vi "Validate Meas Name in Library.vi"(0 "Path":path, 5 "library name":string, 11 "error in (no error)":errorcluster) -> (4 "found":bool, 15 "error out":errorcluster)   [LabVIEW 2021, in "Migrator.lvlib"]
uses:
  Migrator.lvlib
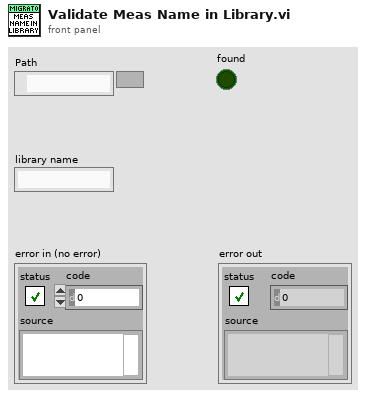
[diagram p1: front panel]
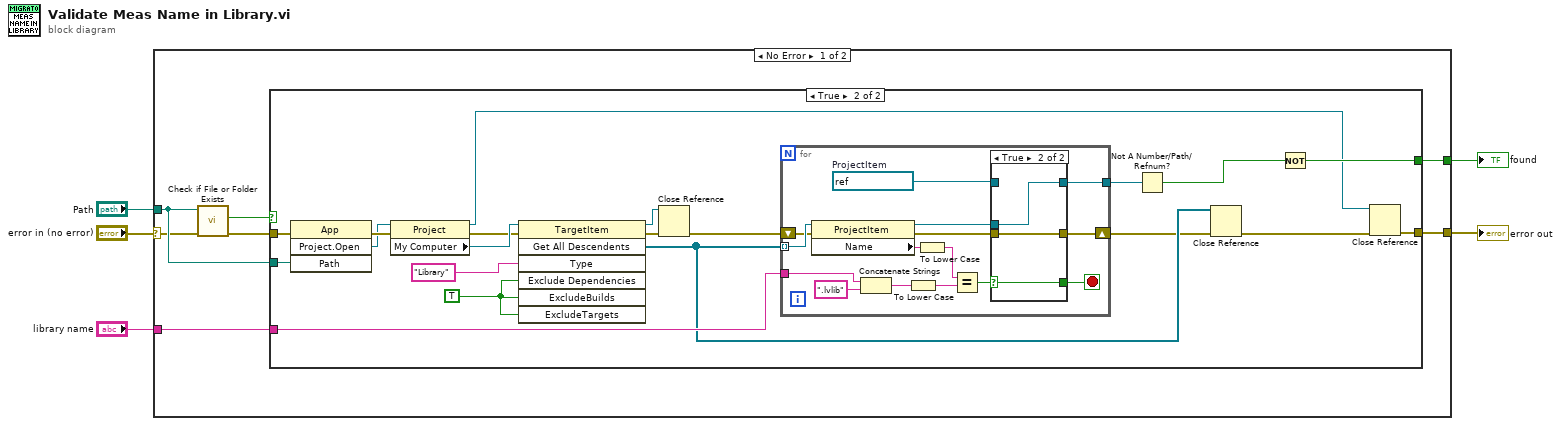
[diagram p0: block diagram]
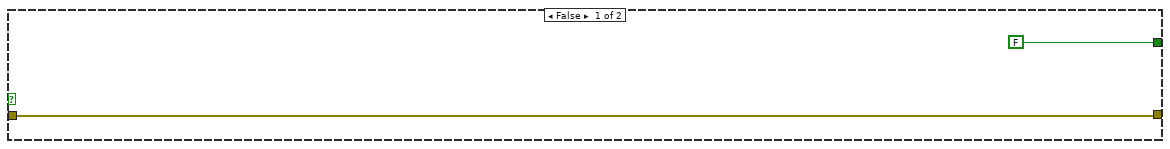
[diagram p2: hidden frame]
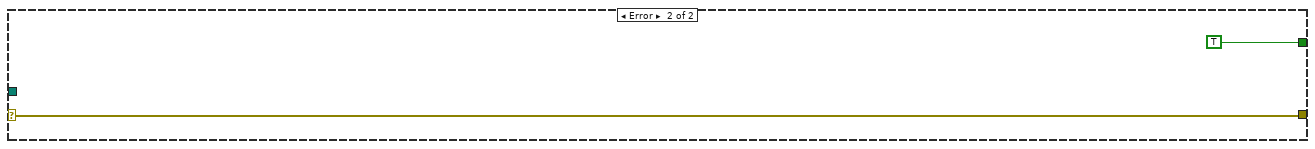
[diagram p4: hidden frame]
diagram:
  n1 = case shown="No Error" "error in (no error)" {
    selector: "error in (no error)" -> [w9 w55]
    tunnel: "library name" -> [w12 _]
    tunnel: "Path" -> [w10 _]
    tunnel: [w11 w55] -> w2
    tunnel: [w7 TRUE] -> w1
    frame No Error {
      n2 = call <vilib>:"Check if File or Folder Exists.vi"("error in (no error)"=w9, "path"=w10) -> ("error out"=w8:errorcluster, "file or folder exists?"=w6:bool)  [unwired: 7 in, 1 out]
      n3 = case shown="True" w6 {
        tunnel: w12 -> [_ w29]
        tunnel: [w13 w22] -> w11
        tunnel: w10 -> [_ w27]
        tunnel: w8 -> [w13 w26]
        tunnel: [FALSE w25] -> w7
        frame False {
        }
        frame True {
          w18 = TRUE ("ExcludeDependencies")
          n4 = invoke class="App" method="Project.Open"(error in=w26, "Path"=w27) -> (error out=w28:errorcluster, "Project:Open"=w23:refnum<vi>)  [unwired: 2 in, 2 out]
          n5 = property class="Project"(reference=w23, error in=w28) -> (reference out=w21:refnum<vi>, error out=w33:errorcluster, "My Computer"=w34:refnum<vi>)
          n6 = invoke class="TargetItem" method="Get All Descendents"(reference=w34, error in=w33, "Type"="Library", "Exclude Dependencies"=w18, "ExcludeBuilds"=w18, "ExcludeTargets"=w18) -> (reference out=w31:refnum<vi>, error out=w32:errorcluster, "All Descendents"=w17:refnum<vi>[])  [unwired: 1 in, 4 out]
          n7 = Close Reference(reference=w31, error in (no error)=w32) -> (error out=w19:errorcluster)
          n8 = for {
            tunnel: w17 -> [w49] mode=indexing
            tunnel: w29 -> [w48]
            shift-right: [w42] -> w15
            shift-left: w19 -> [w46]
            tunnel: [w41] -> w24
            stop <- w36 stop-if-true
            w35 = refnum<vi> refnum  # ProjectItem
            n9 = property class="ProjectItem"(reference=w49, error in=w46) -> (reference out=w44:refnum<vi>, error out=w45:errorcluster, "Name"=w38:string)
            n10 = Concatenate Strings(w48, ".lvlib" ("string")) -> (w40:string)
            n11 = To Lower Case(string=w40) -> (all lower case string=w39:string)
            n12 = To Lower Case(string=w38) -> (all lower case string=w37:string)
            n13 = Equal?(x=w37, y=w39) -> (x = y?=w43:bool)
            n14 = case shown="True" w43 {
              selector: w43 -> [_ w52]
              tunnel: w45 -> [w50 w54]
              tunnel: w44 -> [_ w53]
              tunnel: [w50 w54] -> w42
              tunnel: [w51 w53] -> w41
              tunnel: w35 -> [w51 _]
              tunnel: [_ w52] -> w36
              frame False {
              }
              frame True {
              }
            }
          }
          n15 = Not A Number/Path/Refnum?(number/path/refnum=w24) -> (NaN/Path/Refnum?=w20:bool)
          n16 = Close Reference(reference=w17, error in (no error)=w15) -> (error out=w16:errorcluster)
          n17 = Not(x=w20) -> (.not. x?=w25:bool)
          n18 = Close Reference(reference=w21, error in (no error)=w16) -> (error out=w22:errorcluster)
        }
      }
    }
    frame Error {
    }
  }
  "error out" <- w2
  "found" <- w1
